vi "Controller_Conditioning_vector.vi"(4 "Angular Offset\n(-180 to 180 or 0 to 360)":dbl, 5 "Min Output(0 to 1)":dbl, 6 "n^x(Unbounded)":dbl=2.5 format="%#_13g", 8 "Enum":T1(ring), 9 "Dead Zone(0 to 1)":dbl, 10 "Y(-1 to 1)":dbl, 11 "X(-1 to 1)":dbl) -> (0 "Magnitude":dbl, 1 "Angle":dbl, 2 "Y":dbl, 3 "X":dbl)   [LabVIEW 2017]
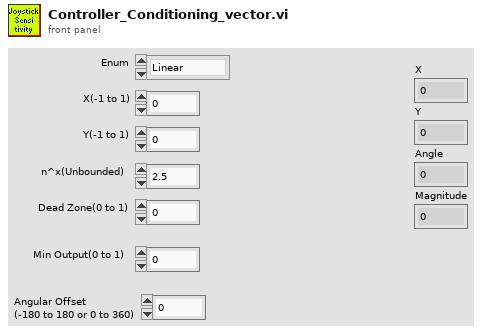
[diagram p1: front panel]
types:
  T1 = enum16{"Linear", "Square  Root", "Square", "n^x"}
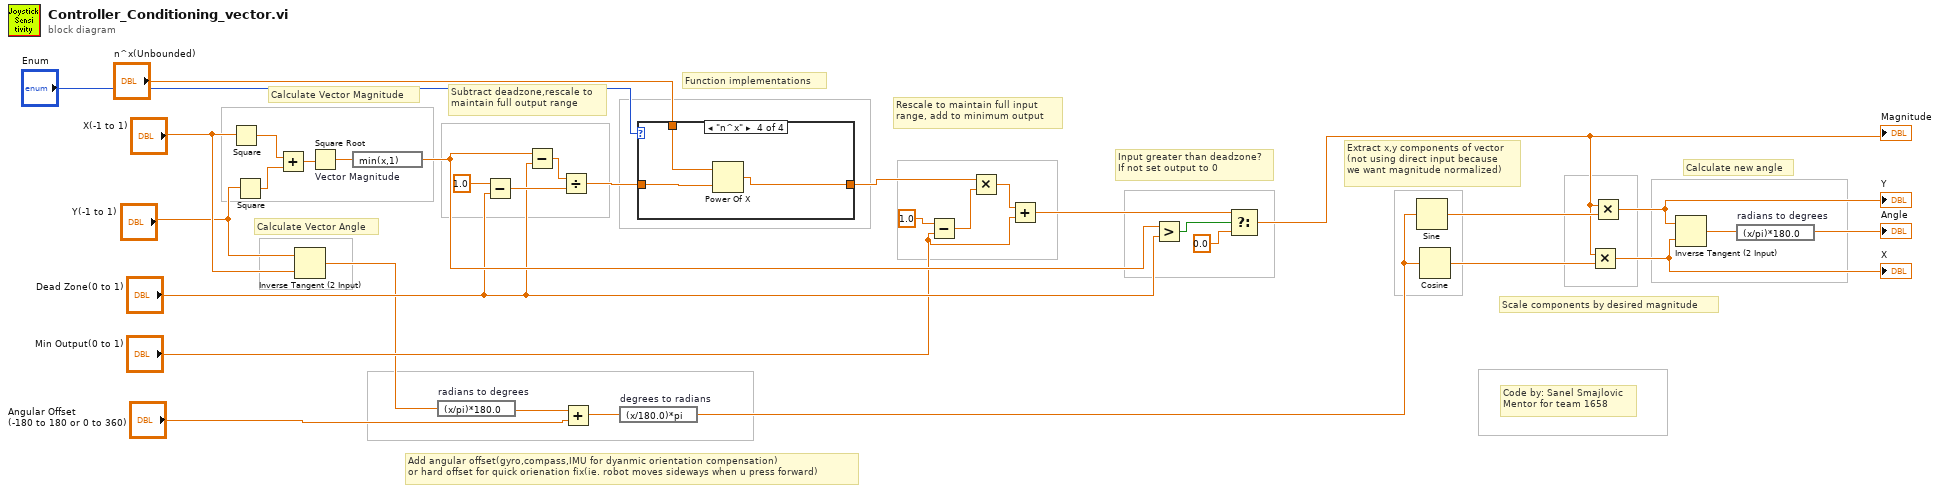
[diagram p0: block diagram]
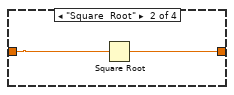
[diagram p3: hidden frame]
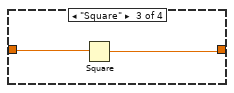
[diagram p4: hidden frame]
diagram:
  # "Add angular offset(gyro,compass,IMU for dyanmic orientation compensation)\nor hard offset for quick orienation fix(ie. robot moves sideways when u press forward)"
  # "Rescale to maintain full input\nrange, add to minimum output"
  # "Subtract deadzone,rescale to \nmaintain full output range"
  # "Code by: Sanel Smajlovic\nMentor for team 1658"
  # "Calculate new angle"
  # "Scale components by desired magnitude"
  # "Extract x,y components of vector\n(not using direct input because\nwe want magnitude normalized)"
  # "Function implementations"
  # "Input greater than deadzone?\nIf not set output to 0"
  # "Calculate Vector Angle"
  # "Calculate Vector Magnitude"
  n1 = Square(x="X(-1 to 1)") -> (x^2=w33:dbl)
  n2 = Square(x="Y(-1 to 1)") -> (x^2=w34:dbl)
  n3 = Add(x=w33, y=w34) -> (x+y=w32:dbl)
  n4 = Inverse Tangent (2 Input)(1:"X(-1 to 1)", 2:"Y(-1 to 1)") -> (0:w9:dbl)
  n5 = Square Root "Vector Magnitude"(x=w32) -> (sqrt(x)=w31:dbl)
  n6 = expression code="min(x,1)"(w31) -> (w22:dbl)
  n7 = expression code="(x/pi)*180.0" "radians to degrees"(w9) -> (w8:dbl)
  n8 = Subtract(x=1.0, y="Dead Zone(0 to 1)") -> (x-y=w19:dbl)
  n9 = Subtract(x=w22, y="Dead Zone(0 to 1)") -> (x-y=w17:dbl)
  n10 = Divide(x=w17, y=w19) -> (x/y=w12:dbl)
  n11 = Add(x=w8, y="Angular Offset\n(-180 to 180 or 0 to 360)") -> (x+y=w6:dbl)
  n12 = expression code="(x/180.0)*pi" "degrees to radians"(w6) -> (w5:dbl)
  n13 = case shown="\"n^x\"" "Enum" {
    tunnel: [w35 w36 w38 w42] -> w11
    tunnel: w12 -> [w35 w37 w39 w41]
    tunnel: "n^x(Unbounded)" -> [_ _ _ w40]
    frame "Linear", Default {
    }
    frame "Square  Root" {
      n14 = Square Root(x=w37) -> (sqrt(x)=w36:dbl)
    }
    frame "Square" {
      n15 = Square(x=w39) -> (x^2=w38:dbl)
    }
    frame "n^x" {
      n16 = Power Of X(1:w41, 2:w40) -> (0:w42:dbl)
    }
  }
  n17 = Subtract(x=1.0, y="Min Output(0 to 1)") -> (x-y=w15:dbl)
  n18 = Multiply(x=w11, y=w15) -> (x*y=w14:dbl)
  n19 = Add(x=w14, y="Min Output(0 to 1)") -> (x+y=w10:dbl)
  n20 = Greater?(x=w22, y="Dead Zone(0 to 1)") -> (0:w24:bool)
  n21 = Select ("Y")(t=w10, s=w24, f=0.0) -> (s? t:f=w3:dbl)
  "Magnitude" <- w3
  n22 = Sine(x=w5) -> (sin(x)=w28:dbl)
  n23 = Cosine(x=w5) -> (cos(x)=w27:dbl)
  n24 = Multiply(x=w3, y=w27) -> (x*y=w4:dbl)
  "X" <- w4
  n25 = Multiply(x=w3, y=w28) -> (x*y=w2:dbl)
  "Y" <- w2
  n26 = Inverse Tangent (2 Input)(1:w4, 2:w2) -> (0:w25:dbl)
  n27 = expression code="(x/pi)*180.0" "radians to degrees"(w25) -> (→"Angle":dbl)
